vi "Line Configuration Dialog.vi"(8 "error in":errorcluster, 9 "engine configuration in":refnum<class "engine configuration.lvclass">, 10 "tag bus configurable plugin module configuration":refnum<class "OPC UA Client configuration.lvclass">, 11 "Line":T3 {"OPC UA Data Type" items=["Boolean"=1, "SByte"=2, "Byte"=3, "Int16"=4, "UInt16"=5, "Int32"=6, "UInt32"=7, "Int64"=8, "UInt64"=9, "Float"=10, "Double"=11, "String"=12, "DateTime"=13, "ByteString"=15, "Array of Boolean"=101, "Array of SByte"=102, "Array of Byte"=103, "Array of Int16"=104, "Array of UInt16"=105, "Array of Int32"=106, "Array of UInt32"=107, "Array of Int64"=108, "Array of UInt64"=109, "Array of Float"=110, "Array of Double"=111, "Array of String"=112, "Array of DateTime"=113, "Array of ByteString"=115]}) -> (0 "error out":errorcluster, 1 "success":bool, 2 "changed":bool, 3 "Mappings out":T2 {"Line"."OPC UA Data Type" items=["Boolean"=1, "SByte"=2, "Byte"=3, "Int16"=4, "UInt16"=5, "Int32"=6, "UInt32"=7, "Int64"=8, "UInt64"=9, "Float"=10, "Double"=11, "String"=12, "DateTime"=13, "ByteString"=15, "Array of Boolean"=101, "Array of SByte"=102, "Array of Byte"=103, "Array of Int16"=104, "Array of UInt16"=105, "Array of Int32"=106, "Array of UInt32"=107, "Array of Int64"=108, "Array of UInt64"=109, "Array of Float"=110, "Array of Double"=111, "Array of String"=112, "Array of DateTime"=113, "Array of ByteString"=115]})   [LabVIEW 2013, in "OPC UA Client editor node.lvclass"]
uses:
  OPC UA Client editor node.lvclass
  module/configuration/Line.ctl
  <vilib>/NI/Tag Bus Module Framework/channel/TBM channel.lvclass
  module/configuration/OPC UA Data Type.ctl
  Mappings.ctl
  Map.ctl
  permissions.ctl
  <vilib>/NI/Module Execution Interface/Engine Configuration/engine configuration.lvclass
  module/configuration/OPC UA Client configuration.lvclass
  <vilib>/NI/Tag Bus Module Framework/channel/TBM channel.lvclass/TBM channel.ctl
  <vilib>/NI/Tag Bus/tag/tag descriptor.lvclass/tag descriptor.ctl
  <vilib>/NI/Configuration Framework/serializable configuration/NISE_CEF_serializable configuration.lvclass/NISE_CEF_serializable configuration.ctl
  <vilib>/NI/Tag Bus/tag/write tag name.vi
  <vilib>/NI/Tag Bus/tag/write data type.vi
  <vilib>/NI/Tag Bus Module Framework/channel/Write channel classification.vi
  <vilib>/NI/Configuration Framework/serializable configuration/Read UID.vi
  <vilib>/NI/Tag Bus Module Framework/channel/Read channel classification.vi
  <vilib>/NI/Tag Bus/tag/read data type.vi
  <vilib>/Utility/LVClass/Get LV Class Name.vi
  <vilib>/NI/Configuration Framework/error generator/NISE_error generator.vi
  <vilib>/NI/Tag Bus/tag/tag descriptor.lvclass
panel:
  in  "Node Path":string
  out "errors":string
  in  "Access Type":T1
  in  "Tag":i32(listbox)
  in  "Data Type":i32(listbox)
  in  "Channel Name":string
  in  "cancel":bool
  in  "ok":bool
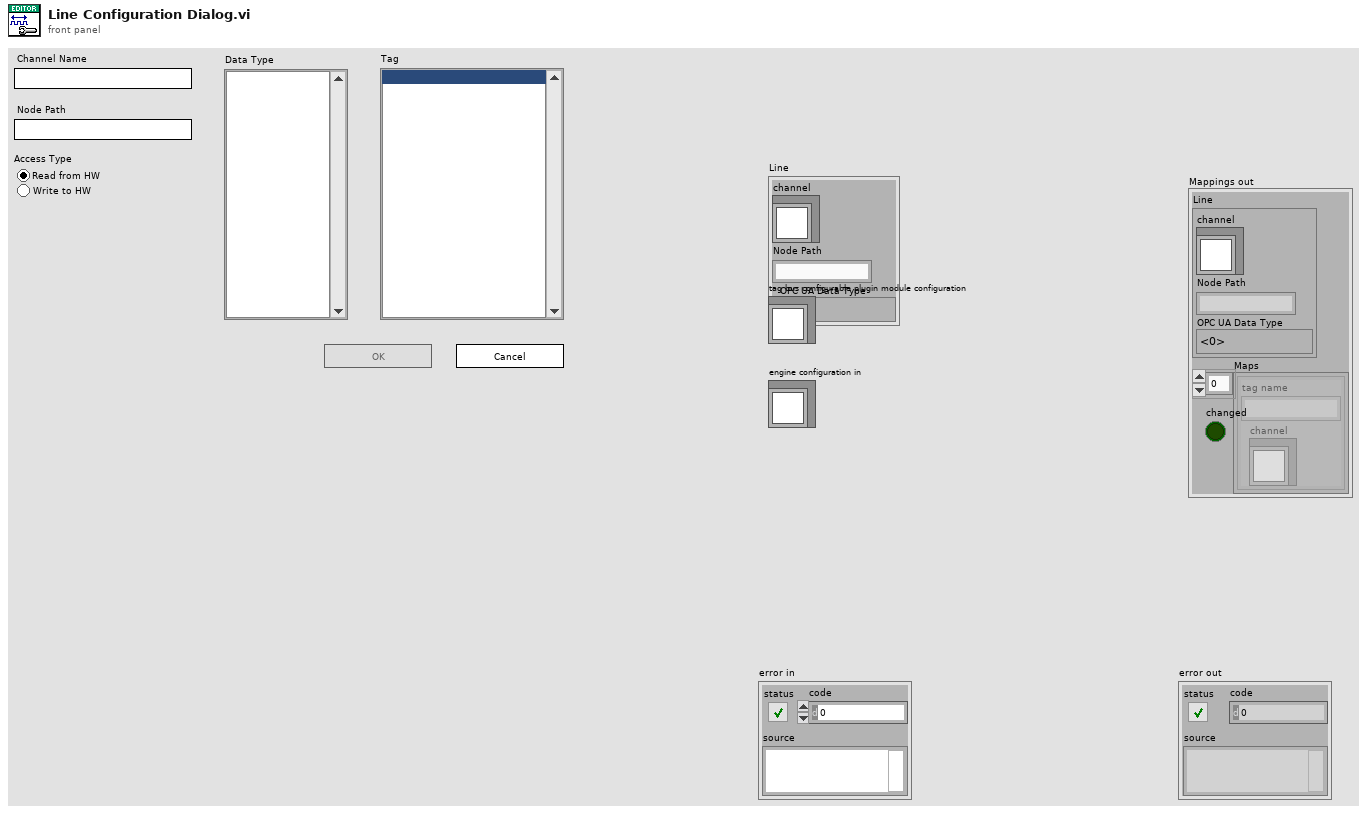
[diagram p1: front panel]
types:
  T1 = typedef "OPC UA Client editor node.lvclass/permissions.ctl" = enum32{"Read from HW", "Write to HW"}
  T2 = typedef "OPC UA Client editor node.lvclass/Mappings.ctl" = cluster{"Line":T3, "Maps":T5[]}
  T3 = typedef "OPC UA Client configuration.lvclass/Line.ctl" = cluster{"channel":refnum<class "TBM channel.lvclass">, "Node Path":string, "OPC UA Data Type":T4}
  T4 = typedef "OPC UA Client configuration.lvclass/OPC UA Data Type.ctl" = u16
  T5 = typedef "OPC UA Client editor node.lvclass/Map.ctl" = cluster{"channel":refnum<class "TBM channel.lvclass">, "tag name":string}
  T6 = typedef "tag bus.lvlib/tag descriptor.lvclass/Data Type.ctl" = enum16{"Double", "Single", "I64", "I32", "I16", "I8", "U64", "U32", "U16", "U8", "Boolean", "String", "Array of Double", "Array of Single", "Array of I64", "Array of I32", "Array of I16", "Array of I8", "Array of U64", "Array of U32", "Array of U16", "Array of U8", "Array of Boolean", "Array of String"}
  T7 = typedef "TBM channel.lvclass/channel classification.ctl" = enum16{"input data", "output data", "processing parameter", "processing result"}
  T8 = enum8{"Enabled", "Disabled", "Disabled and Grayed Out"}
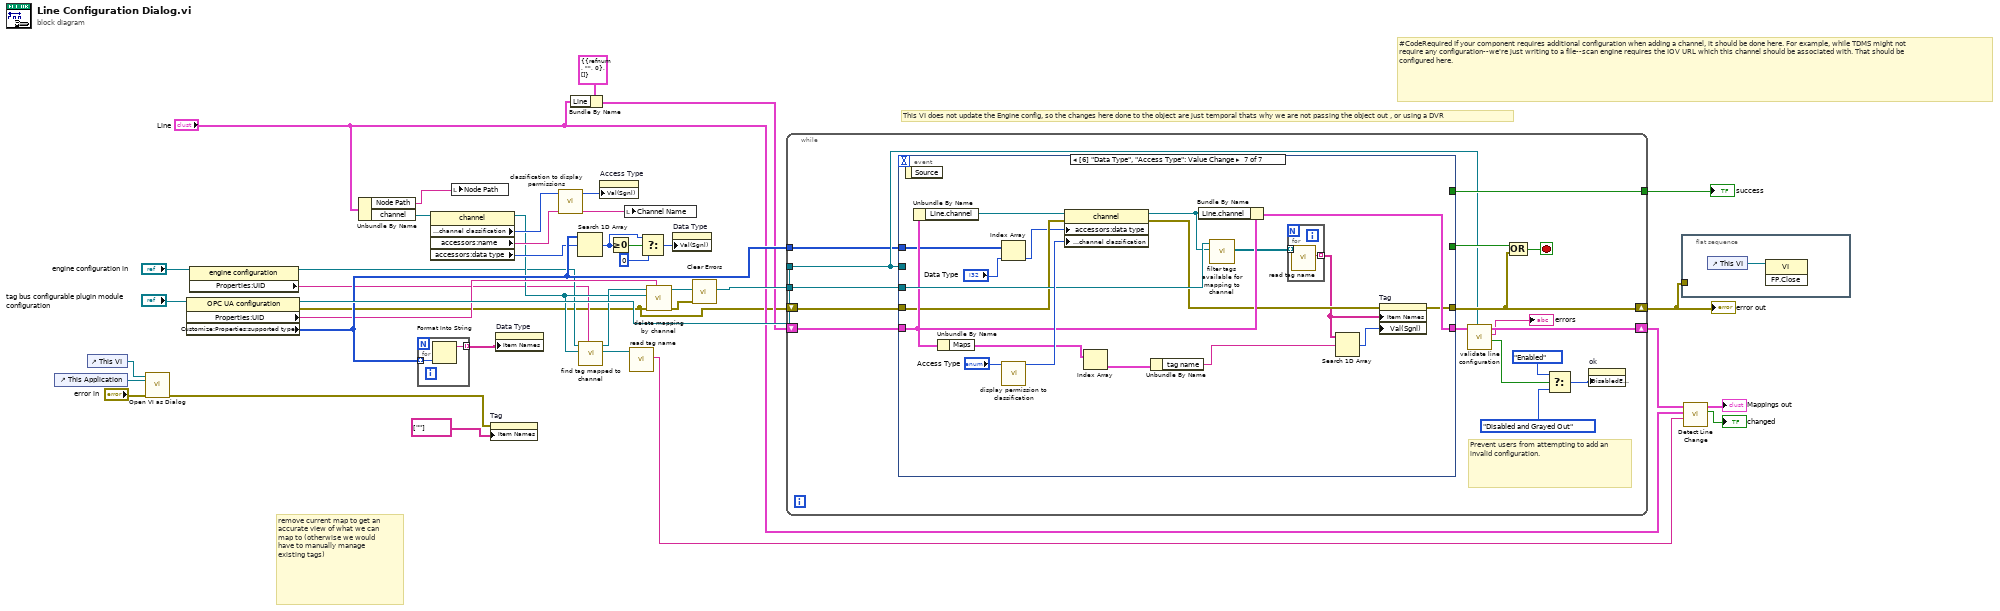
[diagram p0: block diagram]
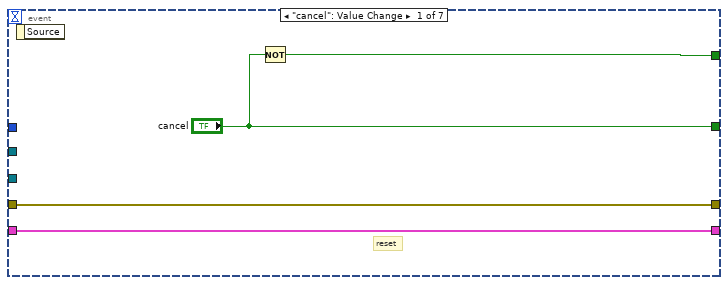
[diagram p2: hidden frame]
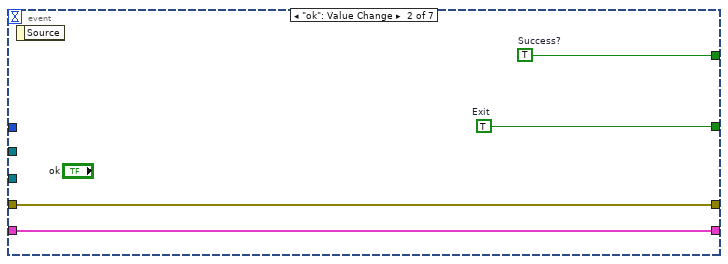
[diagram p3: hidden frame]
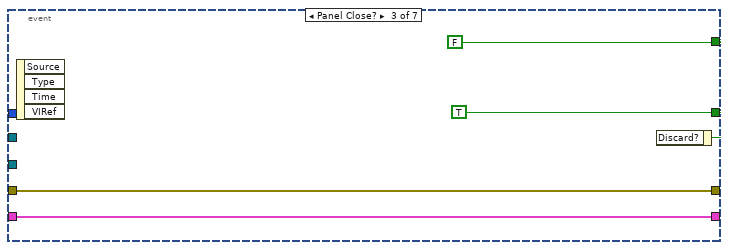
[diagram p4: hidden frame]
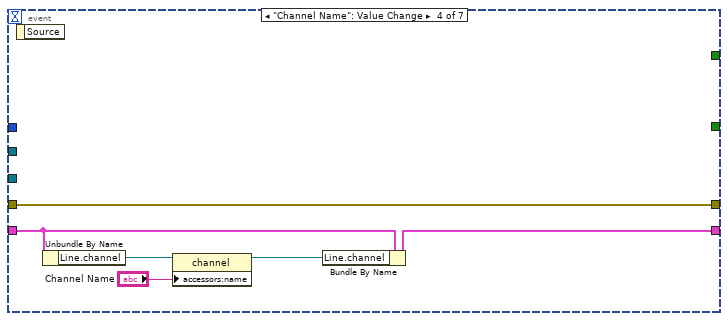
[diagram p5: hidden frame]
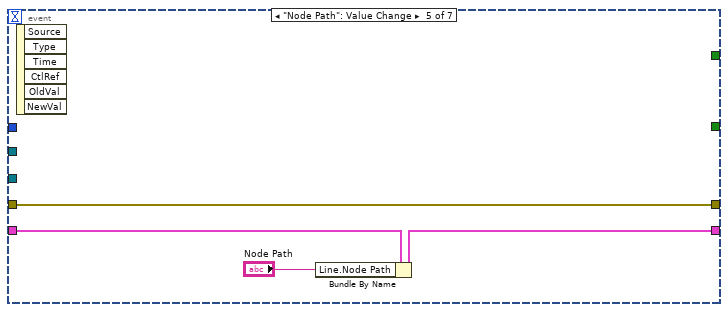
[diagram p6: hidden frame]
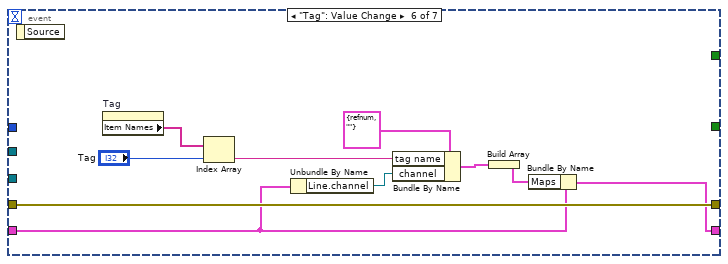
[diagram p7: hidden frame]
diagram:
  # "This VI does not update the Engine config, so the changes here done to the object are just temporal thats why we are not passing the object out , or using a DVR"
  # "remove current map to get an accurate view of what we can map to (otherwise we would have to manually manage existing tags)"
  # "#CodeRequired If your component requires additional configuration when adding a channel, it should be done here. For example, while TDMS might not require any configuration--we're just writing to a file--scan engine requires the IOV URL which this channel should be associated with. That should be configured here."
  n1 = control-ref of="This Application"() -> (w33:refnum<vi>)
  n2 = control-ref of="This VI"() -> (w32:refnum<vi>)
  n3 = call "Open VI as Dialog.vi"("error in (no error)"="error in", "This Application"=w33, "VI in"=w32) -> ("error out"=w15:errorcluster)  [unwired: 8 in]
  n4 = property class="OPC UA configuration"(reference="tag bus configurable plugin module configuration") -> (reference out=w35:refnum<class "OPC UA Client configuration.lvclass">, error out=w1:errorcluster, "Properties:UID"=w27:string, "Customize:Properties:supported types"=w34:T6[])  [unwired: 1 in]
  n5 = property class="engine configuration"(reference="engine configuration in") -> ("Properties:UID"=w2:string)  [unwired: 1 in, 2 out]
  n6 = Unbundle By Name("Line") -> ("Node Path"=w13:string, "channel"=w28:refnum<class "TBM channel.lvclass">)
  n7 = for {
    tunnel: w34 -> [w39] mode=indexing
    tunnel: [w38] -> w26 mode=indexing
    n8 = Format Into String(w39) -> (resulting string=w38:string)  [unwired: 3 in, 1 out]
  }
  n9 = property class="channel"(reference=w28) -> (reference out=w6:refnum<class "TBM channel.lvclass">, "data access:channel classification"=w30:T7, "accessors:name"=w29:string, "accessors:data type"=w19:T6)  [unwired: 1 in, 1 out]
  n10 = local write "Node Path"(w13) -> ()
  n11 = property on="Tag" class="LstBox (strict)"(error in=w15, "Item Names"=string[] [""]) -> ()  [unwired: 1 in, 2 out]
  n12 = property on="Data Type" class="LstBox (strict)"("Item Names"=w26) -> ()  [unwired: 2 in, 2 out]
  n13 = call "classification to display permissions.vi"("channel classification"=w30) -> ("permissions"=w20:T1)  [unwired: 10 in]
  n14 = Bundle By Name(cluster=T2 {"Line"={"channel"=refnum, "Node Path"="", "OPC UA Data Type"=0}, "Maps"=[]} ("Mappings out"), "Line"="Line") -> (w8:T2)
  n15 = Search 1D Array(1D array=w34, element=w19) -> (index of element=w24:i32)  [unwired: 1 in]
  n16 = call <vilib>:"find tag mapped to channel.vi"("owner"=w2, "channel"=w6, "engine configuration in"="engine configuration in") -> ("tag"=w5:refnum<class "tag descriptor.lvclass">, "engine configuration out"=w7:refnum<class "engine configuration.lvclass">)  [unwired: 6 in, 1 out]
  n17 = property on="Access Type" class="RadioBtnsControl (strict)"("Val(Sgnl)"=w20) -> ()  [unwired: 2 in, 2 out]
  n18 = Greater Or Equal To 0?(x=w24) -> (x >= 0?=w25:bool)
  n19 = local write "Channel Name"(w29) -> ()
  n20 = call <vilib>:"read tag name.vi"("system tag in"=w5) -> ("name"=w4:string)  [unwired: 8 in, 2 out]
  n21 = Select(t=w24, s=w25, f=0) -> (s? t:f=w22:i32)
  n22 = call <vilib>:"delete mapping by channel.vi"("owner ID"=w27, "error in"=w1, "channel"=w6, "engine configuration in"=w7) -> ("error out"=w18:errorcluster, "engine configuration out"=w36:refnum<class "engine configuration.lvclass">)  [unwired: 6 in]
  n23 = property on="Data Type" class="LstBox (strict)"("Val(Sgnl)"=w22) -> ()  [unwired: 2 in, 2 out]
  n24 = call <vilib>:"Clear Errors.vi"("error in (no error)"=w18) -> ()  [unwired: 6 in, 1 out]
  n25 = while {
    shift-right: [w47] -> w31
    shift-left: w1 -> [w54]
    tunnel: [w53] -> w37
    shift-right: [w48] -> w12
    shift-left: w8 -> [w50]
    tunnel: w36 -> [w55]
    tunnel: w35 -> [w42]
    tunnel: w34 -> [w41]
    stop <- w51 stop-if-true
    # "Prevent users from attempting to add an invalid configuration."
    n26 = event shown="[6] \"Data Type\", \"Access Type\": Value Change" {
      selector: _ -> [_ _ _ _ _ _ _]
      dyn-events: _ -> [_ _ _ _ _ _ _]
      timeout: _ -> [_ _ _ _ _ _ _]
      tunnel: w55 -> [_ _ _ _ _ _ w104]
      tunnel: w54 -> [w59 w63 w67 w73 w77 w87 w98]
      tunnel: [w59 w63 w67 w73 w77 w87 w93] -> w47
      tunnel: [w58 w60 FALSE _ _ _ _] -> w53
      tunnel: ["cancel" w61 w65 _ _ _ _] -> w52
      tunnel: w50 -> [w56 w62 w64 w71 w76 w81 w102]
      tunnel: [w56 w62 w64 w72 w75 w78 w101] -> w49
      tunnel: w42 -> [_ _ _ _ _ _ _]
      tunnel: w41 -> [_ _ _ _ _ _ w97]
      event "cancel": Value Change {
        # "reset"
        n27 = event-data() -> ()  [unwired: 1 in, 1 out]
        n28 = Not(x="cancel") -> (.not. x?=w58:bool)
      }
      event "ok": Value Change {
        w60 = TRUE  # Success?
        w61 = TRUE  # Exit
        n29 = event-data() -> ()  [unwired: 1 in, 1 out]
      }
      event Panel Close? {
        w65 = TRUE ("cancel")
        n30 = event-data() -> ()  [unwired: 1 in, 4 out]
        n31 = event-data("Discard?"=w65) -> ()  [unwired: 1 in, 1 out]
      }
      event "Channel Name": Value Change {
        n32 = event-data() -> ()  [unwired: 1 in, 1 out]
        n33 = Unbundle By Name(w71) -> ("Line.channel"=w70:refnum<class "TBM channel.lvclass">)
        n34 = property class="channel"(reference=w70, "accessors:name"="Channel Name") -> (reference out=w69:refnum<class "TBM channel.lvclass">)  [unwired: 1 in, 1 out]
        n35 = Bundle By Name(cluster=w71, "Line.channel"=w69) -> (w72:T2)
      }
      event "Node Path": Value Change {
        n36 = event-data() -> ()  [unwired: 1 in, 6 out]
        n37 = Bundle By Name(cluster=w76, "Line.Node Path"="Node Path") -> (w75:T2)
      }
      event "Tag": Value Change {
        n38 = event-data() -> ()  [unwired: 1 in, 1 out]
        n39 = property on="Tag" class="LstBox (strict)"() -> ("Item Names"=w85:string[])  [unwired: 2 in, 2 out]
        n40 = Index Array(array=w85, index="Tag") -> (element=w84:string)
        n41 = Unbundle By Name(w81) -> ("Line.channel"=w82:refnum<class "TBM channel.lvclass">)
        n42 = Bundle By Name(cluster=T5 {"channel"=refnum, "tag name"=""} ("Map"), "tag name"=w84, "channel"=w82) -> (w80:T5)
        n43 = Build Array(w80) -> (w79:T5[])
        n44 = Bundle By Name(cluster=w81, "Maps"=w79) -> (w78:T2)
      }
      event "Data Type": Value Change {
        n45 = event-data() -> ()  [unwired: 1 in, 1 out]
        n46 = Unbundle By Name(w102) -> ("Line.channel"=w106:refnum<class "TBM channel.lvclass">)
        n47 = Unbundle By Name(w102) -> ("Maps"=w90:T5[])
        n48 = Index Array(array=w97, index="Data Type") -> (element=w95:T6)
        n49 = call "display permission to classification.vi"("display permissions"="Access Type") -> ("channel classification"=w105:T7)  [unwired: 10 in]
        n50 = property class="channel"(reference=w106, error in=w98, "accessors:data type"=w95, "data access:channel classification"=w105) -> (reference out=w103:refnum<class "TBM channel.lvclass">, error out=w94:errorcluster)
        n51 = Index Array(array=w90) -> (element=w89:T5)  [unwired: 1 in]
        n52 = Unbundle By Name(w89) -> ("tag name"=w88:string)
        n53 = Bundle By Name(cluster=w102, "Line.channel"=w103) -> (w101:T2)
        n54 = call <vilib>:"filter tags available for mapping to channel.vi"("channel to map to"=w103, "engine configuration in"=w104) -> ("filtered tags"=w100:refnum<class "tag descriptor.lvclass">[])  [unwired: 8 in, 1 out]
        n55 = for {
          tunnel: w100 -> [w108] mode=indexing
          tunnel: [w107] -> w92 mode=indexing
          n56 = call <vilib>:"read tag name.vi"("system tag in"=w108) -> ("name"=w107:string)  [unwired: 8 in, 2 out]
        }
        n57 = Search 1D Array(1D array=w92, element=w88) -> (index of element=w91:i32)  [unwired: 1 in]
        n58 = property on="Tag" class="LstBox (strict)"(error in=w94, "Item Names"=w92, "Val(Sgnl)"=w91) -> (error out=w93:errorcluster)  [unwired: 1 in, 1 out]
      }
    }
    n59 = call "validate line configuration.vi"("module"=w42, "Mappings in"=w49) -> ("valid?"=w46:bool, "errors"=→"errors":string, "Mappings out"=w48:T2)  [unwired: 7 in]
    n60 = Compound Arithmetic op=OR(w52, w47) -> (w51:bool)
    n61 = Select(t=T8."Enabled" ("Disabled"), s=w46, f=T8."Disabled and Grayed Out") -> (s? t:f=w43:T8)
    n62 = property on="ok" class="Bool"("DisabledEnum"=w43) -> ()  [unwired: 2 in, 2 out]
  }
  "error out" <- w31
  "success" <- w37
  n63 = flat-sequence {
    tunnel: w31 -> [_]
    frame #0 {
      n64 = control-ref of="This VI"() -> (w109:refnum<vi>)
      n65 = invoke class="VI" method="FP.Close"(reference=w109) -> ()  [unwired: 2 in, 3 out]
    }
  }
  n66 = call "Detect Line Change.vi"("Original Tag"=w4, "Original Line"="Line", "Mappings In"=w12) -> ("Changed?"=→"changed":bool, "Mappings Out"=→"Mappings out":T2)  [unwired: 7 in]
